vi "Test Handler.vi"(11 "JoystickDevRef":T1={"Device"=enum."USB 1"}) -> ()   [LabVIEW 2019]
uses:
  <vilib>/Rock Robotics/WPI/Joystick/WPI_JoystickDevRef.ctl
  <vilib>/Rock Robotics/WPI/Joystick/WPI_JoystickDeviceEnum.ctl
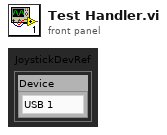
[diagram p1: front panel]
types:
  T1 = typedef "WPI_JoystickDevRef.ctl" = cluster{"Device":T2}
  T2 = typedef "WPI_JoystickDeviceEnum.ctl" = enum16{"USB 0", "USB 1", "USB 2", "USB 3", "USB 4", "USB 5"}
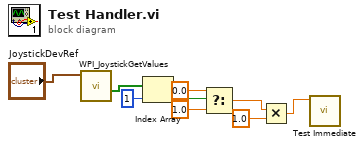
[diagram p0: block diagram]
diagram:
  n1 = call <vilib>:"WPI_JoystickGetValues.vi"("JoystickDevRef"="JoystickDevRef") -> ("Buttons"=w8:bool[])  [unwired: 6 in, 4 out]
  n2 = Index Array(array=w8, index=1) -> (element=w6:bool)
  n3 = Select(t=0.0, s=w6, f=1.0) -> (s? t:f=w2:dbl)
  n4 = Multiply(x=w2, y=1.0) -> (x*y=w1:dbl)
  n5 = call "Test Immediate.vi"("Setpoint"=w1) -> ()  [unwired: 10 in, 1 out]
